vi "AimDetect_R2.vi"(0 "File Path":path=path "C:/mtp/Site_Ne_sch/Projects/AVALANCHE/COMMON/MIMIC Commads/SaveImages/AimSpotGetAimNear_.bmp", 1 "Treshold Range":cluster{"Lower value":sgl, "Upper value":sgl}={"Lower value"=160.0, "Upper value"=255.0}, 7 "error in":errorcluster) -> (19 "Fitted Circle":T1={"Center (Pixels)"={"X"=662.68866, "Y"=339.79785}, "Radius (Pixels)"=48.166488438286514, "Center (Real-World)"={"X"=662.68866, "Y"=339.79785}, "Radius (Real-World)"=48.166488438286514, "Roundness (Real-World)"=0.004982363738023072, "Average Strength"=36.718725718725715, "Average SNR (dB)"=22.939760745828973}, 20 "Coordinate System Out (Set Coordinate System 1)":T4={"Reference System"={"Origin"={"X"=652.9596, "Y"=374.51172}, "Angle (deg)"=0.0, "Axis Reference"=0}, "Measurement System"={"Origin"={"X"=653.0, "Y"=384.0}, "Angle (deg)"=0.0, "Axis Reference"=0}} {"Measurement System"."Axis Reference" items=["Direct", "Indirect"]; "Measurement System"."Angle (deg)" format="%.2f"; "Measurement System"."Origin"."Y" format="%.2f"; "Measurement System"."Origin"."X" format="%.2f"; "Reference System"."Axis Reference" items=["Direct", "Indirect"]; "Reference System"."Angle (deg)" format="%.2f"; "Reference System"."Origin"."Y" format="%.2f"; "Reference System"."Origin"."X" format="%.2f"}, 21 "Nb Circles (Circle Detection 1)":i32, 22 "Circles Data (Circle Detection 1)":T3(array[cluster]), 23 "Number of Particles (Particle Analysis 1)":i32, 24 "Particle Measurements (Pixels) (Particle Analysis 1)":dbl[][](array[numeric]) format="%.2f", 25 "Particle Measurements (Real-World) (Particle Analysis 1)":dbl[][](array[numeric]) format="%.2f", 27 "error out":errorcluster)   [LabVIEW 2014]
uses:
  <vilib>/vision/Measure.llb/Edge Options.ctl
  <vilib>/vision/Measure.llb/Edge Polarity.ctl
  <vilib>/vision/NI_Vision_Development_Module.lvlib
panel:
  out "Circle Found":bool=TRUE
  out "Number of Particles":i32
  out "Image Out":T2(plugin-control)
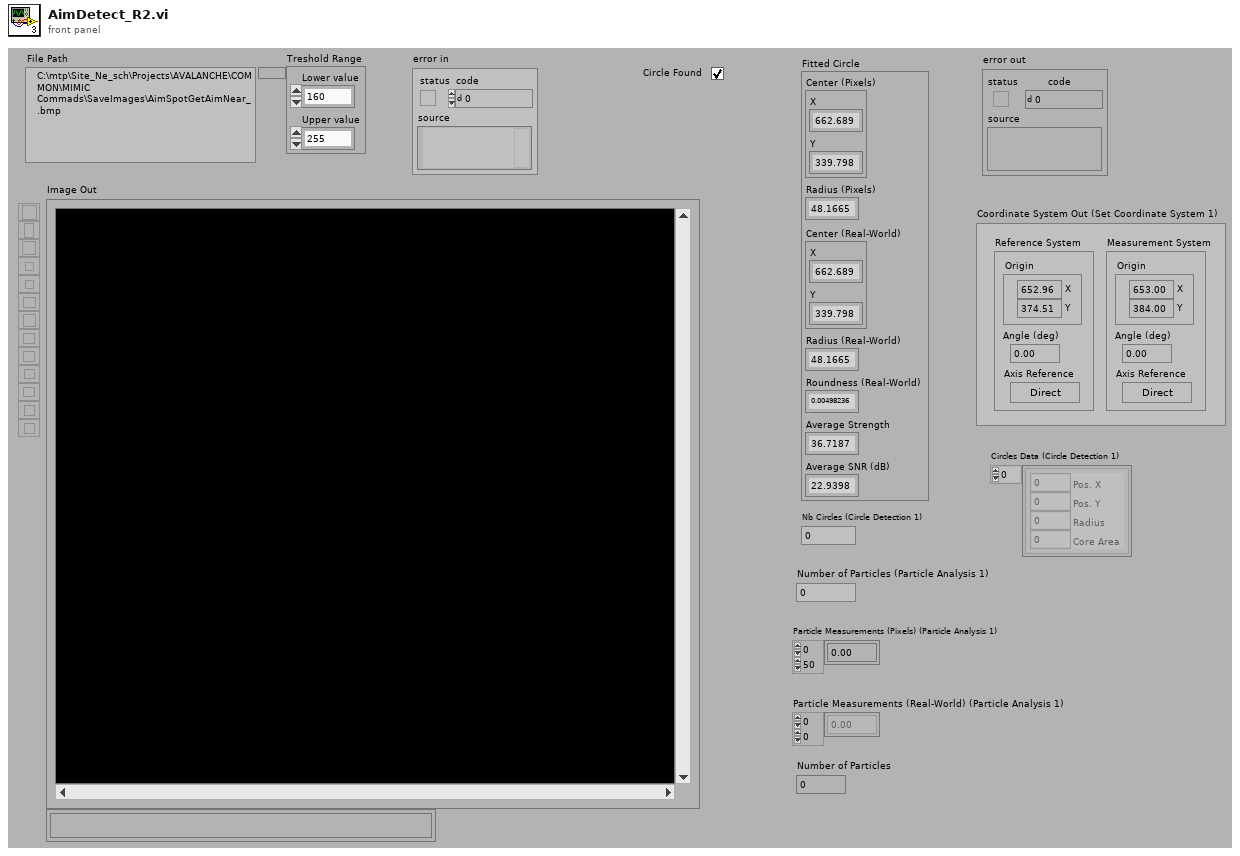
[diagram p1: front panel]
types:
  T1 = cluster{"Center (Pixels)":cluster{"X":sgl, "Y":sgl}, "Radius (Pixels)":dbl, "Center (Real-World)":cluster{"X":sgl, "Y":sgl}, "Radius (Real-World)":dbl, "Roundness (Real-World)":dbl, "Average Strength":dbl, "Average SNR (dB)":dbl}
  T2 = typedef "IMAQ Image.ctl" = refnum<image>
  T3 = cluster{"Pos. X":i32, "Pos. Y":i32, "Radius":i32, "Core Area":i32}[]
  T4 = cluster{"Reference System":cluster{"Origin":cluster{"X":sgl, "Y":sgl}, "Angle (deg)":sgl, "Axis Reference":u32}, "Measurement System":cluster{"Origin":cluster{"X":sgl, "Y":sgl}, "Angle (deg)":sgl, "Axis Reference":u32}}
  T5 = cluster{"Global Rectangle":i32[], "Contours":cluster{"ID":enum32{"External", "Internal"}, "Type":u32, "Coordinates":i32[]}[]}
  T6 = cluster{"Origin":cluster{"X":sgl, "Y":sgl}, "Angle (deg)":sgl, "Axis Reference":u32}
  T7 = enum16{"Reset", "Update Coordinate System", "Get Coordinate System"}
  T8 = typedef "Edge Options.ctl" = cluster{"Edge Polarity":T9, "Kernel Size":u32, "Width":u32, "Minimum Edge Strength":sgl, "Interpolation Type":enum32{"Zero Order", "Bilinear", "Quadratic", "Cubic", "Bilinear Fixed"}, "Data Processing Method":enum32{"Average", "Median"}}
  T9 = typedef "Edge Polarity.ctl" = u32
  T10 = cluster{"Search  Direction":u32, "Edge Options":T8, "Show Search Area":bool, "Show Search Lines":bool, "Show Edges Found":bool, "Show Result":bool, "Search Area Color":u32, "Search Lines Color":u32, "Edge Locations Color":u32, "Result Color":u32, "Overlay Group Name":string}
  T11 = cluster{"Process":enum16{"Get First Edge", "Get First + Last Edge", "Get All Edges", "Get Best Edge"}, "Step Size":i32, "Max Pixel Radius":i32}
  T12 = enum16{"Horizontal Motion", "Vertical Motion", "Horizontal and Vertical Motion", "Horizontal, Vertical and Angular Motion"}
  T13 = typedef "Image Type" = u32
  T14 = typedef "IMAQ Coordinate System" = cluster{"Reference System":cluster{"Origin":cluster{"X":sgl, "Y":sgl}, "Angle (deg)":sgl, "Axis Reference":u32}, "Measurement System":cluster{"Origin":cluster{"X":sgl, "Y":sgl}, "Angle (deg)":sgl, "Axis Reference":u32}}
  T15 = typedef "ROI Descriptor" = cluster{"Global Rectangle":i32[], "Contours":cluster{"ID":enum32{"External", "Internal"}, "Type":u32, "Coordinates":i32[]}[]}
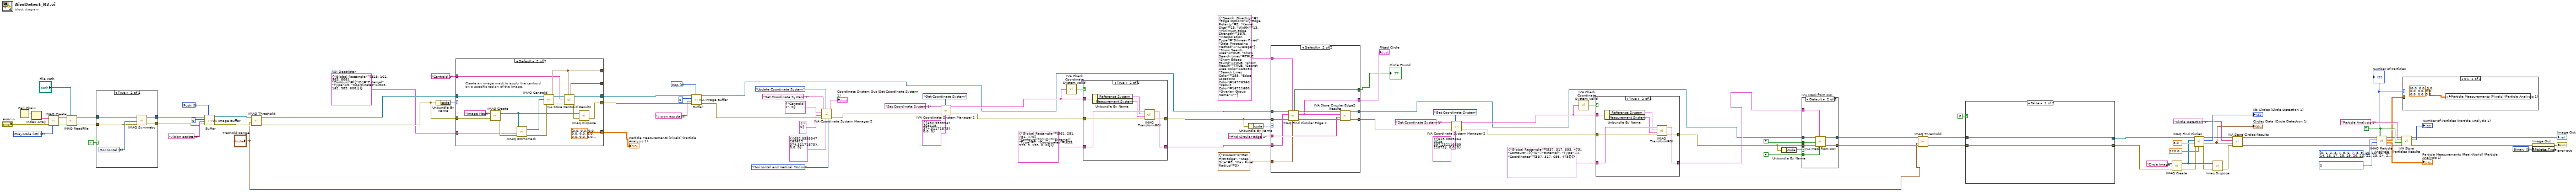
[diagram p0: block diagram]
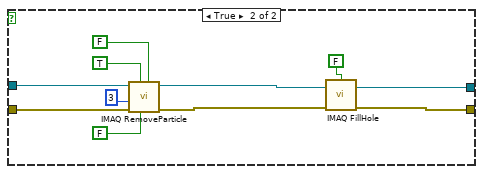
[diagram p2: hidden frame]
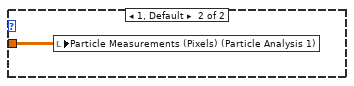
[diagram p4: hidden frame]
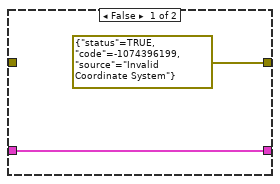
[diagram p6: hidden frame]
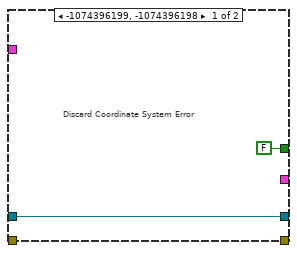
[diagram p7: hidden frame]
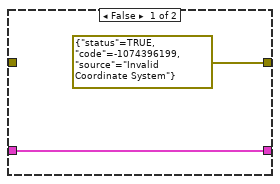
[diagram p8: hidden frame]
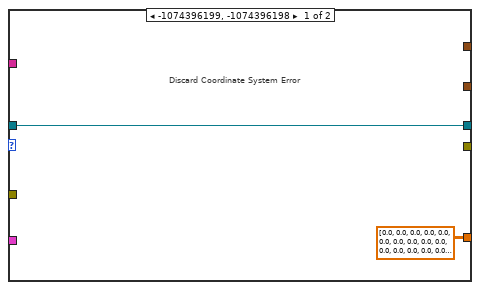
[diagram p9: hidden frame]
diagram:
  w17 = u32 1 items=["Grayscale", "Binary", "Gradient", "Rainbow", "Temperature", "User Defined"] ("Palette")
  w27 = i32[] [] items=["Center of Mass X", "Center of Mass Y", "First Pixel X", "First Pixel Y", "Bounding Rect Left", "Bounding Rect Top", "Bounding Rect Right", "Bounding Rect Bottom", "Max Feret Diameter Start X", "Max Feret Diameter Start Y", "Max Feret Diameter End X", "Max Feret Diameter End Y", "Max Horiz. Segment Length Left", "Max Horiz. Segment Length Right", "Max Horiz. Segment Length Row", "-", "Bounding Rect Width", "Bounding Rect Height", "Bounding Rect Diagonal", "Perimeter", "Convex Hull Perimeter", "Holes' Perimeter", "Max Feret Diameter", "Equivalent Ellipse Major Axis", "Equivalent Ellipse Minor Axis", "Equivalent Ellipse Minor Axis (Feret)", "Equivalent Rect Long Side", "Equivalent Rect Short Side", "Equivalent Rect Diagonal", "Equivalent Rect Short Side (Feret)", "Average Horiz. Segment Length", "Average Vert. Segment Length", "Hydraulic Radius", "Waddel Disk Diameter", "-", "Area", "Holes' Area", "Particle & Holes' Area", "Convex Hull Area", "Image Area", "-", "Number of Holes", "Number of Horiz. Segments", "Number of Vert. Segments", "-", "Orientation", "Max Feret Diameter Orientation", "-", "% Area/Image Area", "% Area/(Particle & Holes' Area)", "Ratio of Equivalent Ellipse Axes", "Ratio of Equivalent Rect Sides", "-", "Elongation Factor", "Compactness Factor", "Heywood Circularity Factor", "Type Factor", "-", "Sum X", "Sum Y", "Sum XX", "Sum XY", "Sum YY", "Sum XXX", "Sum XXY", "Sum XYY", "Sum YYY", "-", "Moment of Inertia XX", "Moment of Inertia XY", "Moment of Inertia YY", "Moment of Inertia XXX", "Moment of Inertia XXY", "Moment of Inertia XYY", "Moment of Inertia YYY", "Norm. Moment of Inertia XX", "Norm. Moment of Inertia XY", "Norm. Moment of Inertia YY", "Norm. Moment of Inertia XXX", "Norm. Moment of Inertia XXY", "Norm. Moment of Inertia XYY", "Norm. Moment of Inertia YYY", "Hu Moment 1", "Hu Moment 2", "Hu Moment 3", "Hu Moment 4", "Hu Moment 5", "Hu Moment 6", "Hu Moment 7"] ("Real-World Measurements")
  w28 = i32[] [0, 1, 2, 3, 4, 5, 6, 7, 8, 9, 10, 11, 12, 13, 14, 16, 17, 18, 19, 20, 21, 22, 23, 24, 25, 26, 27, 28, 29, 30, 31, 32, 33, 35, 36, 37, 38, 39, 41, 42, 43, 45, 46, 48, 49, 50, 51, 53, 54, 55, 56, 58, 59, 60, 61, 62, 63, 64, 65, 66, 68, 69, 70, 71, 72, 73, 74, 75, 76, 77, 78, 79, 80, 81, 82, 83, 84, 85, 86, 87, 88] items=["Center of Mass X", "Center of Mass Y", "First Pixel X", "First Pixel Y", "Bounding Rect Left", "Bounding Rect Top", "Bounding Rect Right", "Bounding Rect Bottom", "Max Feret Diameter Start X", "Max Feret Diameter Start Y", "Max Feret Diameter End X", "Max Feret Diameter End Y", "Max Horiz. Segment Length Left", "Max Horiz. Segment Length Right", "Max Horiz. Segment Length Row", "-", "Bounding Rect Width", "Bounding Rect Height", "Bounding Rect Diagonal", "Perimeter", "Convex Hull Perimeter", "Holes' Perimeter", "Max Feret Diameter", "Equivalent Ellipse Major Axis", "Equivalent Ellipse Minor Axis", "Equivalent Ellipse Minor Axis (Feret)", "Equivalent Rect Long Side", "Equivalent Rect Short Side", "Equivalent Rect Diagonal", "Equivalent Rect Short Side (Feret)", "Average Horiz. Segment Length", "Average Vert. Segment Length", "Hydraulic Radius", "Waddel Disk Diameter", "-", "Area", "Holes' Area", "Particle & Holes' Area", "Convex Hull Area", "Image Area", "-", "Number of Holes", "Number of Horiz. Segments", "Number of Vert. Segments", "-", "Orientation", "Max Feret Diameter Orientation", "-", "% Area/Image Area", "% Area/(Particle & Holes' Area)", "Ratio of Equivalent Ellipse Axes", "Ratio of Equivalent Rect Sides", "-", "Elongation Factor", "Compactness Factor", "Heywood Circularity Factor", "Type Factor", "-", "Sum X", "Sum Y", "Sum XX", "Sum XY", "Sum YY", "Sum XXX", "Sum XXY", "Sum XYY", "Sum YYY", "-", "Moment of Inertia XX", "Moment of Inertia XY", "Moment of Inertia YY", "Moment of Inertia XXX", "Moment of Inertia XXY", "Moment of Inertia XYY", "Moment of Inertia YYY", "Norm. Moment of Inertia XX", "Norm. Moment of Inertia XY", "Norm. Moment of Inertia YY", "Norm. Moment of Inertia XXX", "Norm. Moment of Inertia XXY", "Norm. Moment of Inertia XYY", "Norm. Moment of Inertia YYY", "Hu Moment 1", "Hu Moment 2", "Hu Moment 3", "Hu Moment 4", "Hu Moment 5", "Hu Moment 6", "Hu Moment 7"] ("Pixel Measurements")
  w24 = TRUE ("Connectivity 4/8 (8)")
  w84 = u16 1 items=["Push", "Pop", "Reset"] ("Function")
  w89 = T5 {"Global Rectangle"=[323, 161, 983, 608], "Contours"=[{"ID"=enum."External", "Type"=3, "Coordinates"=[323, 161, 983, 608]}]}  # ROI Descriptor
  w95 = u16 0 items=["Push", "Pop", "Reset"] ("Function")
  w96 = T13 0 items=["Grayscale (U8)", "Grayscale (I16)", "Grayscale (SGL)", "Complex (CSG)", "RGB (U32)", "HSL (U32)", "RGB (U64)", "Grayscale (U16)"] ("Image Type")
  # "Buffer"
  # "Buffer"
  n1 = Call Chain() -> (call chain=w98:string[])
  n2 = Index Array(array=w98) -> (element=w97:string)  [unwired: 1 in]
  n3 = call "IMAQ Create"("Image Name"=w97, "Image Type"=w96, "error in (no error)"="error in") -> ("New Image"=w101:T2, "error out"=w100:errorcluster)  [unwired: 1 in, 1 out]
  n4 = call "IMAQ ReadFile"("File Path"="File Path", "error in (no error)"=w100, "Image"=w101) -> ("error out"=w9:errorcluster, "Image Out"=w10:T2)  [unwired: 2 in, 5 out]
  n5 = case shown="True" TRUE {
    tunnel: [w102 w107] -> w12
    tunnel: [w103 w106] -> w11
    tunnel: w10 -> [w103 w105]
    tunnel: w9 -> [w102 w104]
    frame False {
    }
    frame True {
      w108 = u32 0 items=["Horizontal", "Vertical", "Central", "1st Diagonal", "2nd Diagonal"] ("Type of Symmetry")
      n6 = call "IMAQ Symmetry"("error in (no error)"=w104, "Type of Symmetry"=w108, "Image Src"=w105) -> ("error out"=w107:errorcluster, "Image Dst Out"=w106:T2)  [unwired: 2 in]
    }
  }
  n7 = call <vilib>:"IVA Image Buffer.vi"("Function"=w95, "error in (no error)"=w12, "Prefix"="vision assistant", "Buffer #"=0, "Image In"=w11) -> ("error out"=w14:errorcluster, "Image Out"=w13:T2)  [unwired: 5 out]
  n8 = call "IMAQ Threshold"("error in (no error)"=w14, "Range"="Treshold Range", "Image Src"=w13) -> ("error out"=w92:errorcluster, "Image Dst Out"=w90:T2)  [unwired: 3 in, 4 out]
  n9 = Unbundle By Name(w92) -> ("code"=w87:i32)
  n10 = case shown="Default" w87 {
    tunnel: w92 -> [_ w122]
    tunnel: [_ w121] -> w91
    tunnel: w90 -> [w110 w119]
    tunnel: [w110 w118] -> w86
    tunnel: [_ w117] -> _
    tunnel: [_ w116] -> _
    tunnel: w89 -> [_ w115]
    tunnel: "Centroid 1" ("Step Name") -> [_ w112]
    tunnel: [dbl[][] [[0.0, 0.0, 0.0, 0.0, 0.0, 0.0, 0.0, 0.0, 0.0, 0.0, 0.0, 0.0, 0.0, 0.0, 0.0, 0.0, 0.0, 0.0, 0.0, 0.0, 0.0, 0.0, 0.0, 0.0, 0.0, 0.0, 0.0, 0.0, 0.0, 0.0, 0.0, 0.0, 0.0, 0.0, 0.0, 0.0, 0.0, 0.0, 0.0, 0.0, 0.0, 0.0, 0.0, 0.0, 0.0, 0.0, 0.0, 0.0, 0.0, 0.0, 0.0, 0.0, 0.0, 0.0, 0.0, 0.0, 0.0, 0.0, 0.0, 0.0, 0.0, 0.0, 0.0, 0.0, 0.0, 0.0, 0.0, 0.0, 0.0, 0.0, 0.0, 0.0, 0.0, 0.0, 0.0, 0.0, 0.0, 0.0, 0.0, 0.0, 0.0, 0.0, 0.0, 0.0, 0.0, 0.0, 0.0, 0.0, 0.0, 0.0, 0.0, 0.0, 0.0, 0.0, 0.0, 0.0, 0.0, 0.0, 0.0, 0.0, 0.0]] ("Particle Measurements (Pixels) (Particle Analysis 1)") dbl[][] [[0.0, 0.0, 0.0, 0.0, 0.0, 0.0, 0.0, 0.0, 0.0, 0.0, 0.0, 0.0, 0.0, 0.0, 0.0, 0.0, 0.0, 0.0, 0.0, 0.0, 0.0, 0.0, 0.0, 0.0, 0.0, 0.0, 0.0, 0.0, 0.0, 0.0, 0.0, 0.0, 0.0, 0.0, 0.0, 0.0, 0.0, 0.0, 0.0, 0.0, 0.0, 0.0, 0.0, 0.0, 0.0, 0.0, 0.0, 0.0, 0.0, 0.0, 0.0, 0.0, 0.0, 0.0, 0.0, 0.0, 0.0, 0.0, 0.0, 0.0, 0.0, 0.0, 0.0, 0.0, 0.0, 0.0, 0.0, 0.0, 0.0, 0.0, 0.0, 0.0, 0.0, 0.0, 0.0, 0.0, 0.0, 0.0, 0.0, 0.0, 0.0, 0.0, 0.0, 0.0, 0.0, 0.0, 0.0, 0.0, 0.0, 0.0, 0.0, 0.0, 0.0, 0.0, 0.0, 0.0, 0.0, 0.0, 0.0, 0.0, 0.0]] ("Particle Measurements (Pixels) (Particle Analysis 1)")] -> w7
    frame -1074396199, -1074396198 {
      # "Discard Coordinate System Error"
    }
    frame Default {
      # "Create an image mask to apply the centroid\non a specific region of the image."
      n11 = call "IMAQ Create"("Image Name"="Image Mask", "error in (no error)"=w122) -> ("New Image"=w125:T2, "error out"=w124:errorcluster)  [unwired: 2 in, 1 out]
      n12 = call "IMAQ ROIToMask"("error in (no error)"=w124, "ROI Descriptor"=w115, "Image"=w125) -> ("error out"=w120:errorcluster, "Image Out"=w123:T2)  [unwired: 2 in, 2 out]
      n13 = call "IMAQ Centroid"("error in (no error)"=w120, "Image Mask"=w123, "Image"=w119) -> ("error out"=w114:errorcluster, "Centroid"=w117:cluster{"X Centroid":sgl, "Y Centroid":sgl})  [unwired: 1 out]
      n14 = call <vilib>:"IVA Store Centroid Results.vi"("Centroid in"=w117, "error in (no error)"=w114, "Step Name"=w112, "Image in"=w119) -> ("error out"=w113:errorcluster, "Image dup"=w118:T2, "Calibrated Centroid"=w116:cluster{"X":sgl, "Y":sgl})  [unwired: 5 out]
      n15 = call "Imaq Dispose"("Image"=w125, "error in (no error)"=w113) -> ("error out"=w121:errorcluster)  [unwired: 1 in, 3 out]
    }
  }
  "Particle Measurements (Pixels) (Particle Analysis 1)" <- w7
  n16 = call <vilib>:"IVA Image Buffer.vi"("Function"=w84, "error in (no error)"=w91, "Prefix"="vision assistant", "Buffer #"=0, "Image In"=w86) -> ("error out"=w85:errorcluster, "Image Out"=w65:T2)  [unwired: 5 out]
  n17 = call <vilib>:"IVA Coordinate System Manager 2.vi"("Mode"=T12."Horizontal and Vertical Motion", "Reference System"=T6 {"Origin"={"X"=652.9596, "Y"=374.51172}, "Angle (deg)"=0.0, "Axis Reference"=0}, "Function"=T7."Update Coordinate System", "error in (no error)"=w85, "Angle ID"=cluster{"GUID":string, "Index":i32} {"GUID"="", "Index"=0}, "Origin ID"=cluster{"GUID":string, "Index":i32} {"GUID"="Centroid 1", "Index"=0}, "Coordinate System Name"="Set Coordinate System 1") -> ("error out"=w75:errorcluster, "Coordinate System Out"=→"Coordinate System Out (Set Coordinate System 1)":T14)  [unwired: 3 out]
  n18 = call <vilib>:"IVA Coordinate System Manager 2.vi"("Reference System"=T6 {"Origin"={"X"=652.9596, "Y"=374.51172}, "Angle (deg)"=0.0, "Axis Reference"=0}, "Function"=T7."Get Coordinate System", "error in (no error)"=w75, "Coordinate System Name"="Set Coordinate System 1") -> ("error out"=w71:errorcluster, "Coordinate System Out"=w67:T14)  [unwired: 3 in, 3 out]
  n19 = call <vilib>:"IVA Check Coordinate System Valid.vi"("Coordinate System"=w67) -> ("Valid?"=w66:bool)
  n20 = case shown="True" w66 {
    tunnel: T5 {"Global Rectangle"=[561, 281, 751, 470], "Contours"=[{"ID"=enum."External", "Type"=7, "Coordinates"=[655, 375, 9, 155, 0, 0]}]} ("ROI Descriptor") -> [w127 w135]
    tunnel: [w127 w132] -> w62
    tunnel: [errorcluster {"status"=TRUE, "code"=-1074396199, "source"="Invalid Coordinate System"} ("error out") w131] -> w68
    tunnel: w67 -> [_ w130]
    tunnel: w71 -> [_ w129]
    frame False {
    }
    frame True {
      n21 = Unbundle By Name(w130) -> ("Reference System"=w134:T6, "Measurement System"=w133:T6)
      n22 = call "IMAQ TransformROI"("error in (no error)"=w129, "New Reference"=w133, "Base Reference"=w134, "ROI Descriptor"=w135) -> ("error out"=w131:errorcluster, "ROI Descriptor out"=w132:T15)  [unwired: 6 out]
    }
  }
  n23 = Unbundle By Name(w68) -> ("code"=w61:i32)
  n24 = case shown="Default" w61 {
    tunnel: T10 {"Search  Direction"=1, "Edge Options"={"Edge Polarity"=2, "Kernel Size"=13, "Width"=13, "Minimum Edge Strength"=35.0, "Interpolation Type"=enum."Bilinear Fixed", "Data Processing Method"=enum."Average"}, "Show Search Area"=TRUE, "Show Search Lines"=TRUE, "Show Edges Found"=TRUE, "Show Result"=TRUE, "Search Area Color"=65280, "Search Lines Color"=255, "Edge Locations Color"=16776960, "Result Color"=16711680, "Overlay Group Name"=""} ("Options") -> [_ w139]
    tunnel: w65 -> [w137 w149]
    tunnel: w68 -> [_ w148]
    tunnel: [_ w146] -> w64
    tunnel: [w137 w144] -> w48
    tunnel: "Find Circular Edge 1" ("Step Name") -> [_ w143]
    tunnel: w62 -> [_ w142]
    tunnel: T11 {"Process"=enum."Get First Edge", "Step Size"=3, "Max Pixel Radius"=3} ("Circle Fit Options") -> [_ w141]
    tunnel: [_ w140] -> w5
    tunnel: [FALSE ("Circle Found") w138] -> w3
    frame -1074396199, -1074396198 {
      # "Discard Coordinate System Error"
    }
    frame Default {
      n25 = call "IMAQ Find Circular Edge 2"("Circle Fit Options"=w141, "Options"=w139, "error in (no error)"=w148, "ROI Descriptor"=w142, "Image"=w149) -> ("error out"=w147:errorcluster, "Fitted Circle"=w140:T1, "Image Out"=w145:T2, "Circle Found"=w138:bool)  [unwired: 1 in, 2 out]
      n26 = call <vilib>:"IVA Store Circular Edge2 Results.vi"("error in (no error)"=w147, "Step Name"=w143, "Fitted Circle"=w140, "Image in"=w145) -> ("error out"=w146:errorcluster, "Image dup"=w144:T2)  [unwired: 2 in, 4 out]
    }
  }
  "Fitted Circle" <- w5
  "Circle Found" <- w3
  n27 = call <vilib>:"IVA Coordinate System Manager 2.vi"("Reference System"=T6 {"Origin"={"X"=615.08057, "Y"=397.23212}, "Angle (deg)"=0.0, "Axis Reference"=0}, "Function"=T7."Get Coordinate System", "error in (no error)"=w64, "Coordinate System Name"="Set Coordinate System 1") -> ("error out"=w56:errorcluster, "Coordinate System Out"=w52:T14)  [unwired: 3 in, 3 out]
  n28 = call <vilib>:"IVA Check Coordinate System Valid.vi"("Coordinate System"=w52) -> ("Valid?"=w51:bool)
  n29 = case shown="True" w51 {
    tunnel: T5 {"Global Rectangle"=[537, 317, 695, 475], "Contours"=[{"ID"=enum."External", "Type"=4, "Coordinates"=[537, 317, 695, 475]}]} ("ROI Descriptor") -> [w150 w158]
    tunnel: [w150 w155] -> w50
    tunnel: [errorcluster {"status"=TRUE, "code"=-1074396199, "source"="Invalid Coordinate System"} ("error out") w154] -> w53
    tunnel: w52 -> [_ w153]
    tunnel: w56 -> [_ w152]
    frame False {
    }
    frame True {
      n30 = Unbundle By Name(w153) -> ("Reference System"=w157:T6, "Measurement System"=w156:T6)
      n31 = call "IMAQ TransformROI"("error in (no error)"=w152, "New Reference"=w156, "Base Reference"=w157, "ROI Descriptor"=w158) -> ("error out"=w154:errorcluster, "ROI Descriptor out"=w155:T15)  [unwired: 6 out]
    }
  }
  n32 = Unbundle By Name(w53) -> ("code"=w45:i32)
  n33 = case "IVA Mask from ROI" shown="Default" w45 {
    tunnel: w50 -> [_ w166]
    tunnel: FALSE ("Shrink") -> [_ w165]
    tunnel: w48 -> [w159 w164]
    tunnel: w53 -> [_ w163]
    tunnel: [_ w162] -> w47
    tunnel: [w159 w161] -> w44
    tunnel: FALSE ("Out / In") -> [_ w160]
    frame -1074396199, -1074396198 {
      # "Discard\nCoordinate\nSystem\nError"
    }
    frame Default {
      n34 = call <vilib>:"IVA Mask from ROI.vi"("Shrink"=w165, "ROI Descriptor"=w166, "error in (no error)"=w163, "Out / In"=w160, "Image Src"=w164) -> ("error out"=w162:errorcluster, "Image Out"=w161:T2)  [unwired: 5 out]
    }
  }
  n35 = call "IMAQ Threshold"("error in (no error)"=w47, "Range"="Treshold Range", "Image Src"=w44) -> ("error out"=w43:errorcluster, "Image Dst Out"=w42:T2)  [unwired: 3 in, 4 out]
  n36 = case shown="False" FALSE {
    tunnel: w43 -> [w167 w179]
    tunnel: w42 -> [w168 w174]
    tunnel: [w167 w170] -> w41
    tunnel: [w168 w169] -> w31
    frame False {
    }
    frame True {
      n37 = call "IMAQ RemoveParticle"("Connectivity 4/8 (8)"=FALSE, "Low Pass/High Pass (Low)"=FALSE, "Square/Hexa (Square)"=TRUE, "error in (no error)"=w179, "Number of Erosion"=3, "Image Src"=w174) -> ("error out"=w173:errorcluster, "Image Dst Out"=w171:T2)  [unwired: 1 in, 3 out]
      n38 = call "IMAQ FillHole"("error in (no error)"=w173, "Image Src"=w171, "Connectivity 4/8 (8)"=FALSE) -> ("error out"=w170:errorcluster, "Image Dst Out"=w169:T2)  [unwired: 1 in, 2 out]
    }
  }
  n39 = call "IMAQ Create"("Image Name"="Circle Image", "error in (no error)"=w41) -> ("New Image"=w36:T2, "error out"=w35:errorcluster)  [unwired: 2 in, 1 out]
  n40 = call "IMAQ Find Circles"("Max Radius"=sgl 120.0, "error in (no error)"=w35, "Min Radius"=sgl 3.0, "Image Dst"=w36, "Image Src"=w31) -> ("error out"=w34:errorcluster, "Circles Data"=w29:T3, "Nb Circles"=→"Nb Circles (Circle Detection 1)":i32)  [unwired: 4 out]
  "Circles Data (Circle Detection 1)" <- w29
  n41 = call "Imaq Dispose"("Image"=w36, "error in (no error)"=w34) -> ("error out"=w33:errorcluster)  [unwired: 1 in, 3 out]
  n42 = call <vilib>:"IVA Store Circles Results.vi"("error in (no error)"=w33, "Circles Data"=w29, "Step Name"="Circle Detection 1", "Image in"=w31) -> ("error out"=w32:errorcluster, "Image dup"=w25:T2)  [unwired: 6 out]
  n43 = call "IMAQ Particle Analysis"("Connectivity 4/8 (8)"=w24, "error in (no error)"=w32, "Real-World Measurements"=w27, "Pixel Measurements"=w28, "Image"=w25) -> ("error out"=w21:errorcluster, "Particle Measurements (Real-World)"=→"Particle Measurements (Real-World) (Particle Analysis 1)":dbl[][], "Particle Measurements (Pixels)"=w8:dbl[][], "Image Out (duplicate)"=w23:T2, "Number of Particles"=w6:i32)  [unwired: 2 out]
  "Number of Particles" <- w6
  n44 = call <vilib>:"IVA Store Particles Results.vi"("error in (no error)"=w21, "Connectivity 4/8 (8)"=w24, "Step Name"="Particle Analysis 1", "Image in"=w23) -> ("error out"=w20:errorcluster, "Number of Particles"=→"Number of Particles (Particle Analysis 1)":i32, "Image dup"=→"Image Out":T2)  [unwired: 5 out]
  n45 = case shown="0" w6 {
    tunnel: w8 -> [_ w181]
    frame 0 {
      n46 = local write "Particle Measurements (Pixels) (Particle Analysis 1)"(dbl[][] [[0.0, 0.0, 0.0, 0.0, 0.0, 0.0, 0.0, 0.0, 0.0, 0.0, 0.0, 0.0, 0.0, 0.0, 0.0, 0.0, 0.0, 0.0, 0.0, 0.0, 0.0, 0.0, 0.0, 0.0, 0.0, 0.0, 0.0, 0.0, 0.0, 0.0, 0.0, 0.0, 0.0, 0.0, 0.0, 0.0, 0.0, 0.0, 0.0, 0.0, 0.0, 0.0, 0.0, 0.0, 0.0, 0.0, 0.0, 0.0, 0.0, 0.0, 0.0, 0.0, 0.0, 0.0, 0.0, 0.0, 0.0, 0.0, 0.0, 0.0, 0.0, 0.0, 0.0, 0.0, 0.0, 0.0, 0.0, 0.0, 0.0, 0.0, 0.0, 0.0, 0.0, 0.0, 0.0, 0.0, 0.0, 0.0, 0.0, 0.0, 0.0, 0.0, 0.0, 0.0, 0.0, 0.0, 0.0, 0.0, 0.0, 0.0, 0.0, 0.0, 0.0, 0.0, 0.0, 0.0, 0.0, 0.0, 0.0, 0.0, 0.0]] ("Particle Measurements (Pixels) (Particle Analysis 1)")) -> ()
    }
    frame 1, Default {
      n47 = local write "Particle Measurements (Pixels) (Particle Analysis 1)"(w181) -> ()
    }
  }
  n48 = property on="Image Out" class="ImageControl"(error in=w20, "Palette:Palette Type"=w17) -> (error out=→"error out":errorcluster)  [unwired: 1 in, 1 out]
